vi "IntersectLines.vi"(10 "Line2D_2":T2, 11 "Line2D_1":T2) -> (2 "Intersect?":bool, 3 "Intersection":T1)   [LabVIEW 2014]
uses:
  TypeDefs/Line2D.ctl
  TypeDefs/Point2DwSlope.ctl
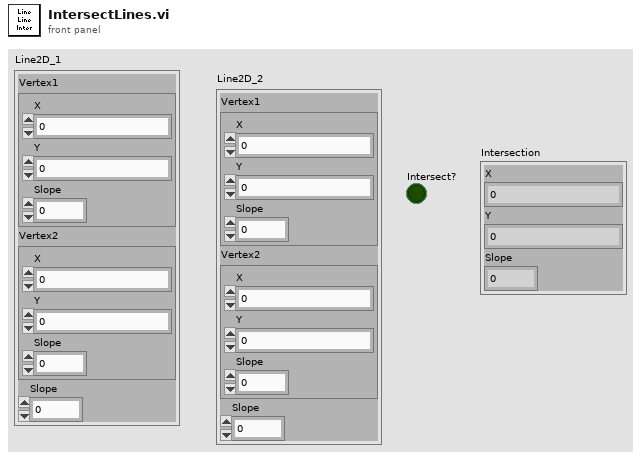
[diagram p1: front panel]
types:
  T1 = typedef "Point2DwSlope.ctl" = cluster{"X":sgl, "Y":sgl, "Slope":dbl}
  T2 = typedef "Line2D.ctl" = cluster{"Vertex1":T1, "Vertex2":T1, "Slope":dbl}
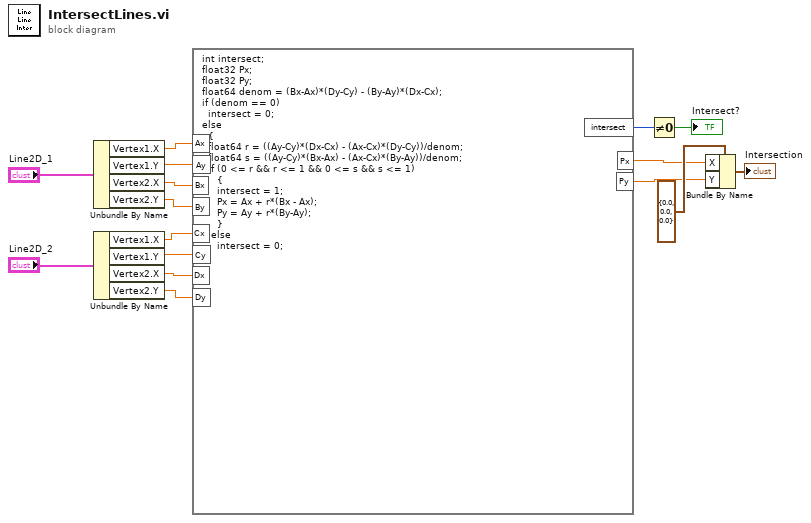
[diagram p0: block diagram]
diagram:
  n1 = Unbundle By Name("Line2D_1") -> ("Vertex1.X"=w14:sgl, "Vertex1.Y"=w13:sgl, "Vertex2.X"=w12:sgl, "Vertex2.Y"=w11:sgl)
  n2 = Unbundle By Name("Line2D_2") -> ("Vertex1.X"=w10:sgl, "Vertex1.Y"=w9:sgl, "Vertex2.X"=w8:sgl, "Vertex2.Y"=w7:sgl)
  n3 = formula code="int intersect;\nfloat32 Px;\nfloat32 Py;\nfloat64 denom = (Bx-Ax)*(Dy-Cy) - (By-Ay)*(Dx-Cx);\nif (denom == 0)\n  intersect = 0;\nelse\n  {\n  float64 r = ((Ay-Cy)*(Dx-Cx) - (Ax-Cx)*(Dy-Cy))/denom;\n  float64 s = ((Ay-Cy)*(Bx-Ax) - (Ax-Cx)*(By-Ay))/denom;\n  if (0 <= r && r <= 1 && 0 <= s && s <= 1)\n     {\n     intersect = 1;\n     Px = Ax + r*(Bx - Ax);\n     Py = Ay + r*(By-Ay);\n     }\n   else\n     intersect = 0;\n}"("Ax"=w14, "Ay"=w13, "Bx"=w12, "By"=w11, "Cx"=w10, "Cy"=w9, "Dx"=w8, "Dy"=w7) -> ("intersect"=w6:i32, "Px"=w3:sgl, "Py"=w2:sgl)
  n4 = Not Equal To 0?(x=w6) -> (x != 0?=→"Intersect?":bool)
  n5 = Bundle By Name(cluster=T1 {"X"=0.0, "Y"=0.0, "Slope"=0.0} ("Point2D"), "X"=w3, "Y"=w2) -> (→"Intersection":T1)
